vi "SetTableHeaderJustify.vi"(5 "列ヘッダ位置":enum16{"Left", "Center", "Right"}[](array[ring]), 7 "列ヘッダ":string[](array[string]), 8 "error in (no error)":errorcluster caption="エラー入力（エラーなし）", 9 "行ヘッダ位置":enum16{"Left", "Center", "Right"}[](array[ring]), 10 "行ヘッダ":string[](array[string]), 11 "Table入力":refnum<vi>) -> (0 "error out":errorcluster caption="エラー出力", 3 "Table入力(copy)":refnum<vi>)   [LabVIEW 2014]
uses:
  <vilib>/Utility/miscctls.llb/LVRowAndColumnTypeDef.ctl
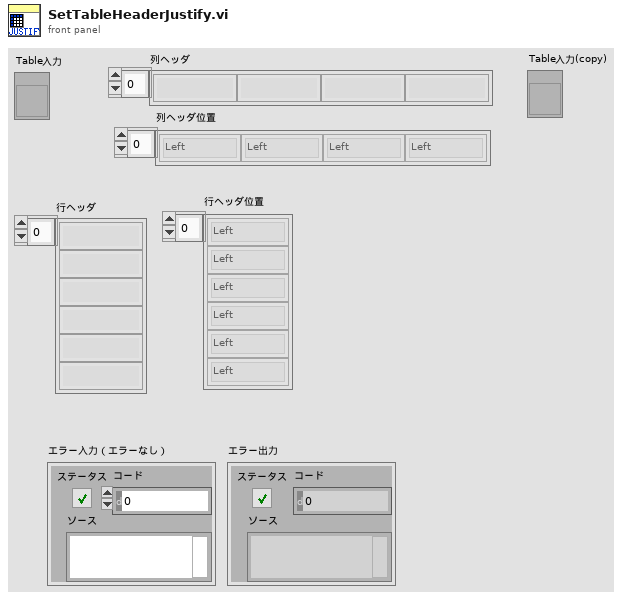
[diagram p1: front panel]
types:
  T1 = typedef "LVRowAndColumnTypeDef.ctl" = cluster{"Row":i32, "Column":i32}
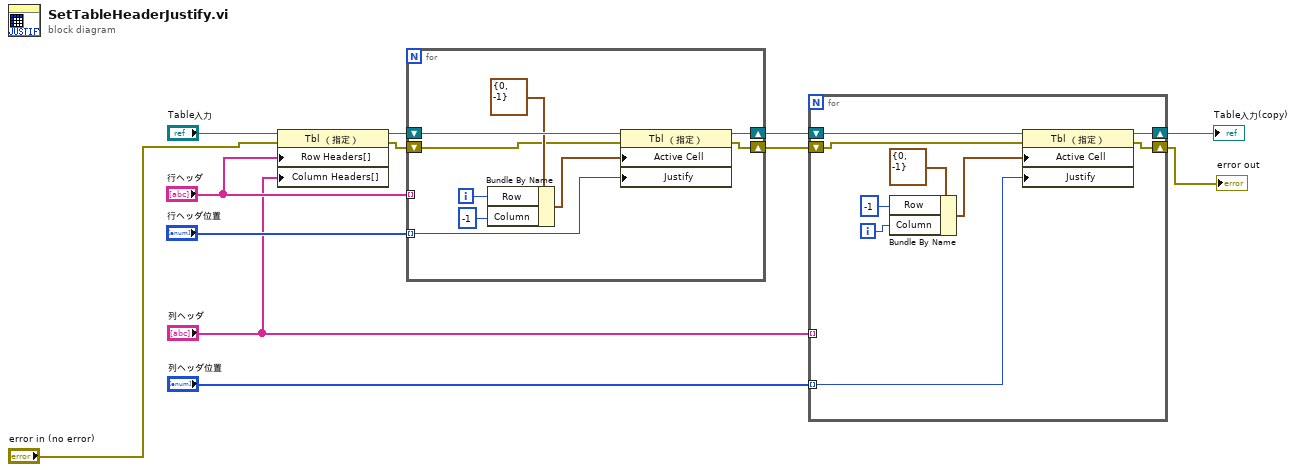
[diagram p0: block diagram]
diagram:
  n1 = property class="Tbl （指定）"(reference="Table入力", error in="error in (no error)", "Row Headers[]"="行ヘッダ", "Column Headers[]"="列ヘッダ") -> (reference out=w11:refnum<vi>, error out=w3:errorcluster)
  n2 = for {
    tunnel: "行ヘッダ" -> [_] mode=indexing
    tunnel: "行ヘッダ位置" -> [w16] mode=indexing
    shift-right: [w15] -> w6
    shift-left: w11 -> [w21]
    shift-right: [w13] -> w2
    shift-left: w3 -> [w14]
    i -> [w18]
    n3 = Bundle By Name(cluster=T1 {"Row"=0, "Column"=-1} ("アクティブセル:アクティブセル"), "Row"=w18, "Column"=-1) -> (w19:T1)
    n4 = property class="Tbl （指定）"(reference=w21, error in=w14, "Active Cell"=w19, "Justify"=w16) -> (reference out=w15:refnum<vi>, error out=w13:errorcluster)
  }
  n5 = for {
    tunnel: "列ヘッダ" -> [_] mode=indexing
    tunnel: "列ヘッダ位置" -> [w25] mode=indexing
    shift-right: [w24] -> w5
    shift-left: w6 -> [w30]
    shift-right: [w22] -> w1
    shift-left: w2 -> [w23]
    i -> [w26]
    n6 = Bundle By Name(cluster=T1 {"Row"=0, "Column"=-1} ("アクティブセル:アクティブセル"), "Row"=-1 ("Column"), "Column"=w26) -> (w28:T1)
    n7 = property class="Tbl （指定）"(reference=w30, error in=w23, "Active Cell"=w28, "Justify"=w25) -> (reference out=w24:refnum<vi>, error out=w22:errorcluster)
  }
  "Table入力(copy)" <- w5
  "error out" <- w1
